vi "Pos_Resolution.vi"(1 "Target":dbl, 2 "Current":dbl) -> (0 "Within resolution?":bool)   [LabVIEW 2010]
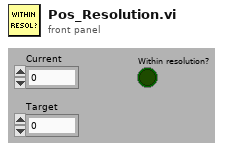
[diagram p1: front panel]
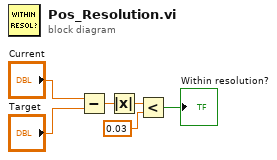
[diagram p0: block diagram]
diagram:
  n1 = Subtract(x="Current", y="Target") -> (x-y=w4:dbl)
  n2 = Absolute Value(x=w4) -> (abs(x)=w3:dbl)
  n3 = Less?(x=w3, y=0.03) -> (x < y?=→"Within resolution?":bool)
